vi "Control Window.vi"(8 "error in (no error)":errorcluster, 10 "Function":T1(ring)=enum."SW_SHOW", 11 "window refnum":T2) -> (0 "error out":errorcluster, 3 "dup window refnum":T2)   [LabVIEW 2020, in "MacroAssert.lvlib" / "Win Util.lvlib"]
doc: "This VI acts as a \"Master\" for various VIs that use the LVPostMessage function in the LVWUTIL.DLL library. This is basically just the PostMessage API function with a WM_SYSCOMMAND message, but also does some additional checking for the existance of the targeted window."
uses:
  Win Util.lvlib
  Window Refnum.ctl
  user32.dll
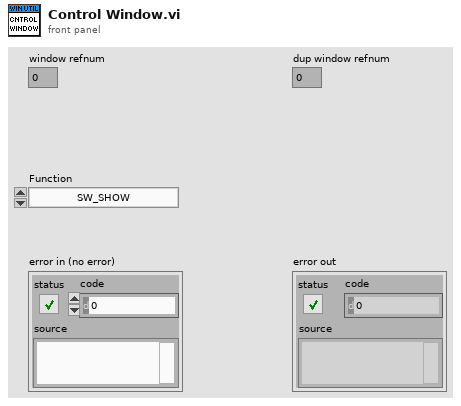
[diagram p1: front panel]
types:
  T1 = enum8{"SW_HIDE", "SW_SHOWNORMAL", "SW_SHOWMINIMIZED", "SW_MAXIMIZE", "SW_SHOWNOACTIVATE", "SW_SHOW", "SW_MINIMIZE", "SW_SHOWMINNOACTIVATE", "SW_SHOWNA", "SW_RESTORE", "SW_SHOWDEFAULT", "SW_FORCEMINIMIZE"}
  T2 = typedef "MacroAssert.lvlib/Win Util.lvlib/Window Refnum.ctl" = u64
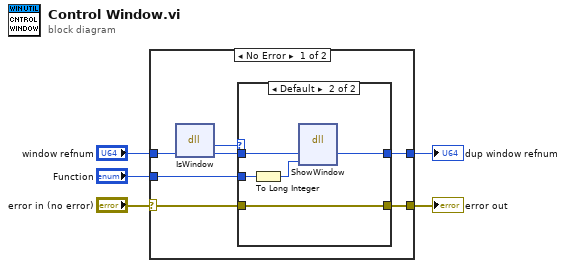
[diagram p0: block diagram]
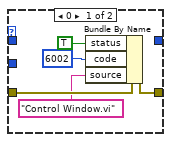
[diagram p2: hidden frame]
diagram:
  n1 = case shown="No Error" "error in (no error)" {
    selector: "error in (no error)" -> [w9 w23]
    tunnel: [w8 w23] -> w3
    tunnel: "window refnum" -> [w12 w24]
    tunnel: [w11 w24] -> w2
    tunnel: "Function" -> [w6 _]
    frame No Error {
      n2 = dll-call lib="user32.dll" fn="IsWindow"("hWnd"=w12) -> ("IsWindow?"=w10:i32, "hWnd"=w7:u64)  [unwired: 3 in, 2 out]
      n3 = case shown="Default" w10 {
        tunnel: w7 -> [_ w22]
        tunnel: [_ w21] -> w11
        tunnel: w9 -> [w16 w20]
        tunnel: [w15 w20] -> w8
        tunnel: w6 -> [_ w19]
        frame 0 {
          n4 = Bundle By Name(cluster=w16, "status"=TRUE ("show call chain? (False)"), "code"=6002, "source"="Control Window.vi") -> (w15:errorcluster)
        }
        frame Default {
          n5 = To Long Integer(number=w19) -> (32bit integer=w18:i32)
          n6 = dll-call lib="user32.dll" fn="ShowWindow"("hWnd"=w22, "function"=w18) -> ("hWnd"=w21:u64)  [unwired: 4 in, 3 out]
        }
      }
    }
    frame Error {
    }
  }
  "error out" <- w3
  "dup window refnum" <- w2
